vi "AN97005H-Config.vi"(6 "下浮值":string, 7 "上浮值":string, 8 "error in":errorcluster caption="错误输入（无错误）", 9 "频率(0.1HZ)":string, 10 "电压(0.1V)":string, 11 "MyIndex":u8) -> (0 "error out":errorcluster caption="错误输出", 3 "OK?":bool)   [LabVIEW 2015, in "AN97005N.lvlib"]
uses:
  AN97005N.lvlib
  <vilib>/Instr/_visa.llb/VISA Configure Serial Port (Instr).vi
panel:
  out "AC电源":refnum<visa-resource-name>
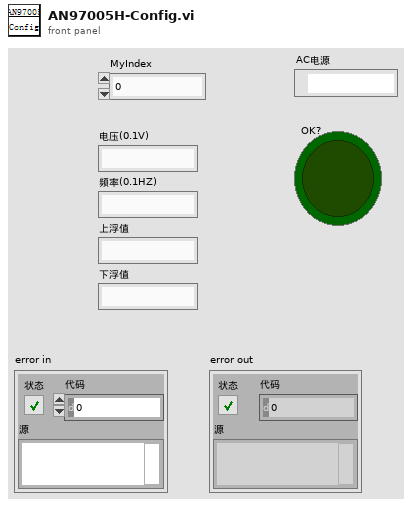
[diagram p1: front panel]
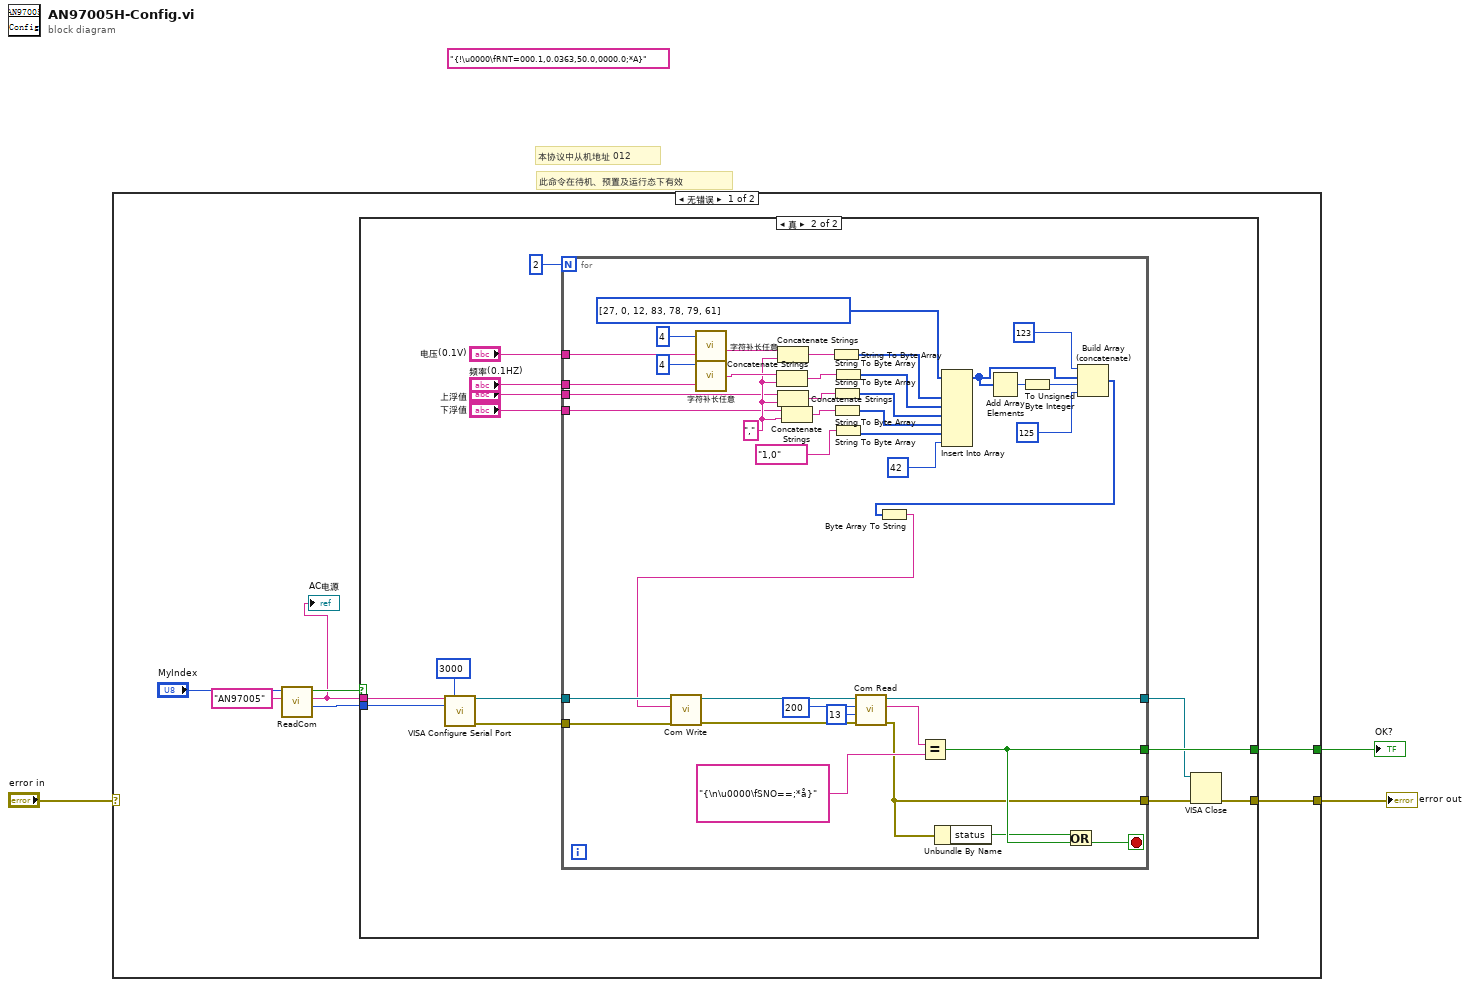
[diagram p0: block diagram]
diagram:
  (unwired) "{!\u0000\fRNT=000.1,0.0363,50.0,0000.0;*A}"
  # "此命令在待机、预置及运行态下有效"
  # "本协议中从机地址 012"
  n1 = case shown="无错误" "error in" {
    selector: "error in" -> [_ w66]
    tunnel: [w10 _] -> w3
    tunnel: [w4 w66] -> w1
    frame No Error {
      n2 = call "ReadCom.vi"("仪器名称"="AN97005", "MyIndex"="MyIndex") -> ("Baudrate"=w6:i32, "COM"=w5:string, "OK?"=w7:bool)  [unwired: 7 in]
      "AC电源" <- w5
      n3 = case shown="真" w7 {
        tunnel: [_ w24] -> w10
        tunnel: [_ w14] -> w4
        tunnel: w5 -> [_ w20]
        tunnel: w6 -> [_ w12]
        frame False {
        }
        frame True {
          n4 = call-poly "VISA Configure Serial Port"("VISA resource name"=w20, "timeout (10sec)"=u32 3000, "baud rate (9600)"=w12) -> ("VISA resource name out"=w22:refnum<visa-resource-name>, "error out"=w15:errorcluster)  [unwired: 11 in]
          n5 = for {
            N: 2 -> [_]
            tunnel: [w58] -> w24
            tunnel: [w32] -> w23
            tunnel: w22 -> [w65]
            tunnel: "电压(0.1V)" -> [w30]
            tunnel: "频率(0.1HZ)" -> [w29]
            tunnel: "上浮值" -> [w28]
            tunnel: "下浮值" -> [w27]
            tunnel: w15 -> [w26]
            tunnel: [w25] -> w13
            stop <- w33 stop-if-true
            w38 = ","
            n6 = call "字符补长任意.vi"("in"=w30, "长度"=u8 4) -> ("out"=w56:string)
            n7 = call "字符补长任意.vi"("in"=w29, "长度"=u8 4) -> ("out"=w54:string)
            n8 = Concatenate Strings(w54, w38) -> (w42:string)
            n9 = Concatenate Strings(w56, w38) -> (w43:string)
            n10 = Concatenate Strings(w28, w38) -> (w41:string)
            n11 = Concatenate Strings(w27, w38) -> (w37:string)
            n12 = String To Byte Array(string=w43) -> (unsigned byte array=w52:u8[])
            n13 = String To Byte Array(string=w41) -> (unsigned byte array=w50:u8[])
            n14 = String To Byte Array(string=w37) -> (unsigned byte array=w49:u8[])
            n15 = String To Byte Array(string=w42) -> (unsigned byte array=w51:u8[])
            n16 = String To Byte Array(string="1,0") -> (unsigned byte array=w35:u8[])
            n17 = Insert Into Array(array=u8[] [27, 0, 12, 83, 78, 79, 61], new element #1=w52, new element #2=w51, new element #3=w50, new element #4=w49, new element #5=w35, new element #6=42) -> (w46:u8[])  [unwired: 1 in]
            n18 = Add Array Elements(numeric array=w46) -> (sum=w48:u8)
            n19 = To Unsigned Byte Integer(number=w48) -> (unsigned 8bit integer=w45:u8)
            n20 = Build Array (concatenate)(123, w46, w45, 125) -> (w40:i32[])
            n21 = Byte Array To String(unsigned byte array=w40) -> (string=w39:string)
            n22 = call "Com Write.vi"("错误输入（无错误）"=w26, "Wbuff"=w39, "VISA In"=w65) -> ("错误输出"=w63:errorcluster, "VISA Out"=w64:refnum<visa-resource-name>)  [unwired: 7 in]
            n23 = call "Com Read.vi"("错误输入（无错误）"=w63, "num"=u32 13, "超时"=u32 200, "VISA In"=w64) -> ("错误输出"=w32:errorcluster, "buff"=w60:string, "VISA Out"=w25:refnum<visa-resource-name>)  [unwired: 5 in]
            n24 = Equal?(x=w60, y="{\n\u0000\fSNO==;*å}" ("Wbuff")) -> (x = y?=w58:bool)
            n25 = Unbundle By Name(w32) -> ("status"=w31:bool)
            n26 = Or(x=w31, y=w58) -> (x .or. y?=w33:bool)
          }
          n27 = VISA Close(VISA resource name=w13, error in (no error)=w23) -> (error out=w14:errorcluster)
        }
      }
    }
    frame Error {
    }
  }
  "OK?" <- w3
  "error out" <- w1
